vi "Day 18-Parse Number.vi"(11 "Data in":string) -> (3 "Data out":i32[][](array[numeric]))   [LabVIEW 2021]
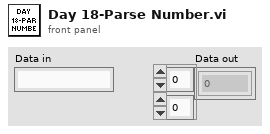
[diagram p1: front panel]
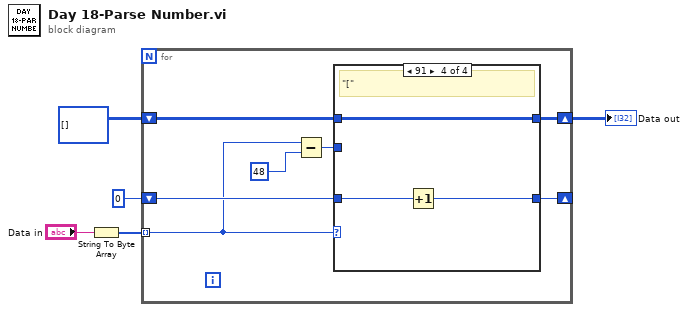
[diagram p0: block diagram]
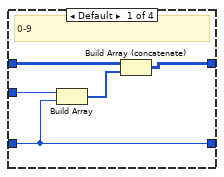
[diagram p2: hidden frame]
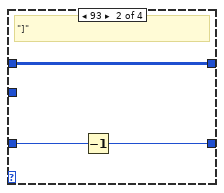
[diagram p3: hidden frame]
diagram:
  n1 = String To Byte Array(string="Data in") -> (unsigned byte array=w1:u8[])
  n2 = for {
    tunnel: w1 -> [w6] mode=indexing
    shift-right: [w11] -> _
    shift-left: 0 -> [w12]
    shift-right: [w7] -> w5
    shift-left: i32[][] [] -> [w10]
    n3 = Subtract(x=w6, y=u8 48) -> (x-y=w8:u8)
    n4 = case shown="91" w6 {
      tunnel: w12 -> [w16 w19 w22 w25]
      tunnel: [w16 w18 w22 w24] -> w11
      tunnel: w10 -> [w15 w20 w21 w23]
      tunnel: w8 -> [w17 _ _ _]
      tunnel: [w13 w20 w21 w23] -> w7
      frame Default {
        # "0-9"
        n5 = Build Array(w17, w16) -> (w14:i32[])
        n6 = Build Array (concatenate)(w15, w14) -> (w13:i32[][])
      }
      frame 93 {
        # "\"]\""
        n7 = Decrement(x=w19) -> (x-1=w18:i32)
      }
      frame 44 {
        # "\",\""
      }
      frame 91 {
        # "\"[\""
        n8 = Increment(x=w25) -> (x+1=w24:i32)
      }
    }
  }
  "Data out" <- w5
